vi "Turn Vision.vi"(0 "Angle from camera":dbl, 1 "AUTO ALIGIN":bool, 5 "From Current Pitch Positon":dbl, 7 "From Joystick V Align":dbl, 9 "Angle Gyro":dbl, 10 "True from shooter":bool, 11 "From joystick Right drive":dbl, 12 "From joystick left drive":dbl) -> (4 "To Left Drive":dbl, 6 "To Corrected Pitch":dbl, 8 "To Joystick V Align":dbl, 14 "True to shooter\n(update position)":bool, 15 "To Right Drive":dbl)   [LabVIEW 2015]
uses:
  <vilib>/Rock Robotics/Network Tables/NT Write Boolean.vi
  <vilib>/Rock Robotics/Network Tables/NT Read Number.vi
  <vilib>/Rock Robotics/Network Tables/NT Read Boolean.vi
panel:
  out "Shoot!":bool
  # "From Controller\nFor Vision"
  # "Inputs to controll vision"
  # "Outputs to control robot"
  # "From Controller for no vision"
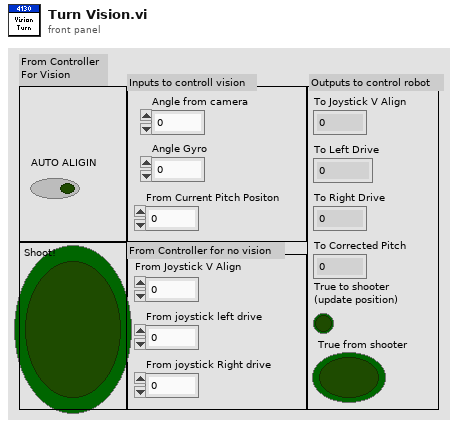
[diagram p1: front panel]
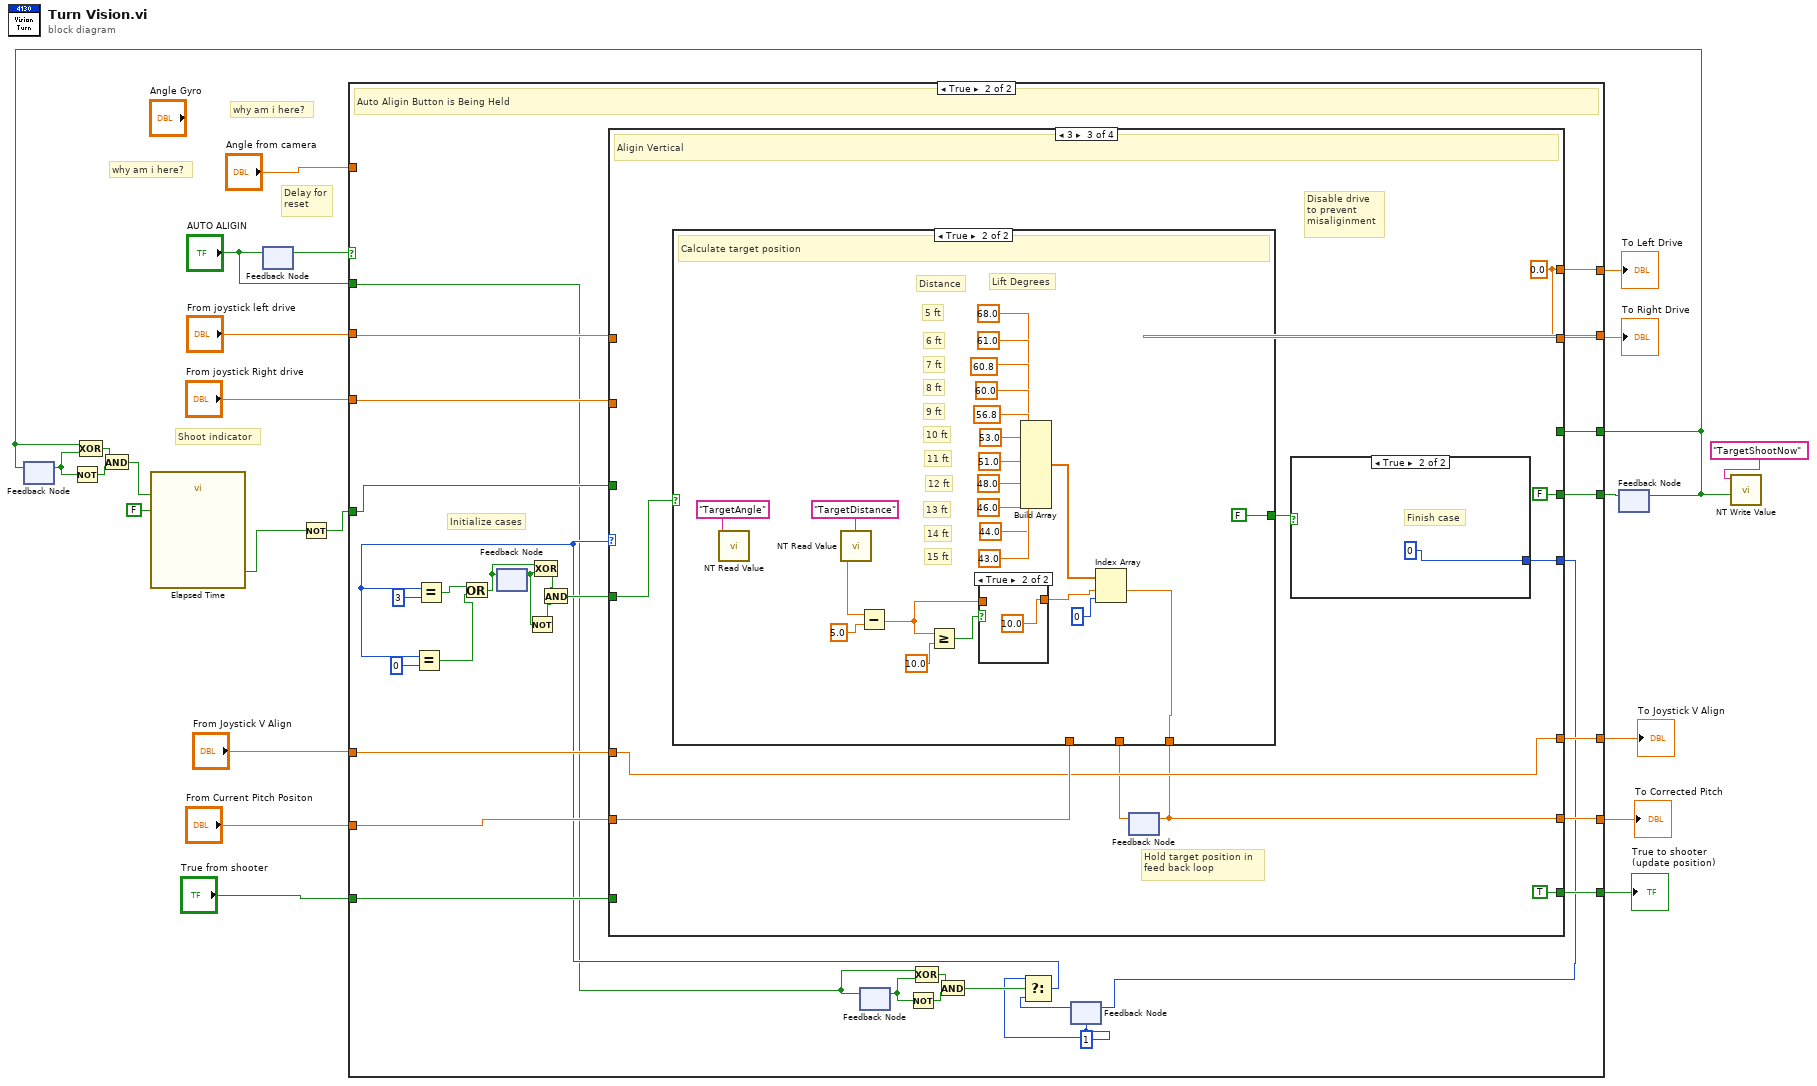
[diagram p0: block diagram]
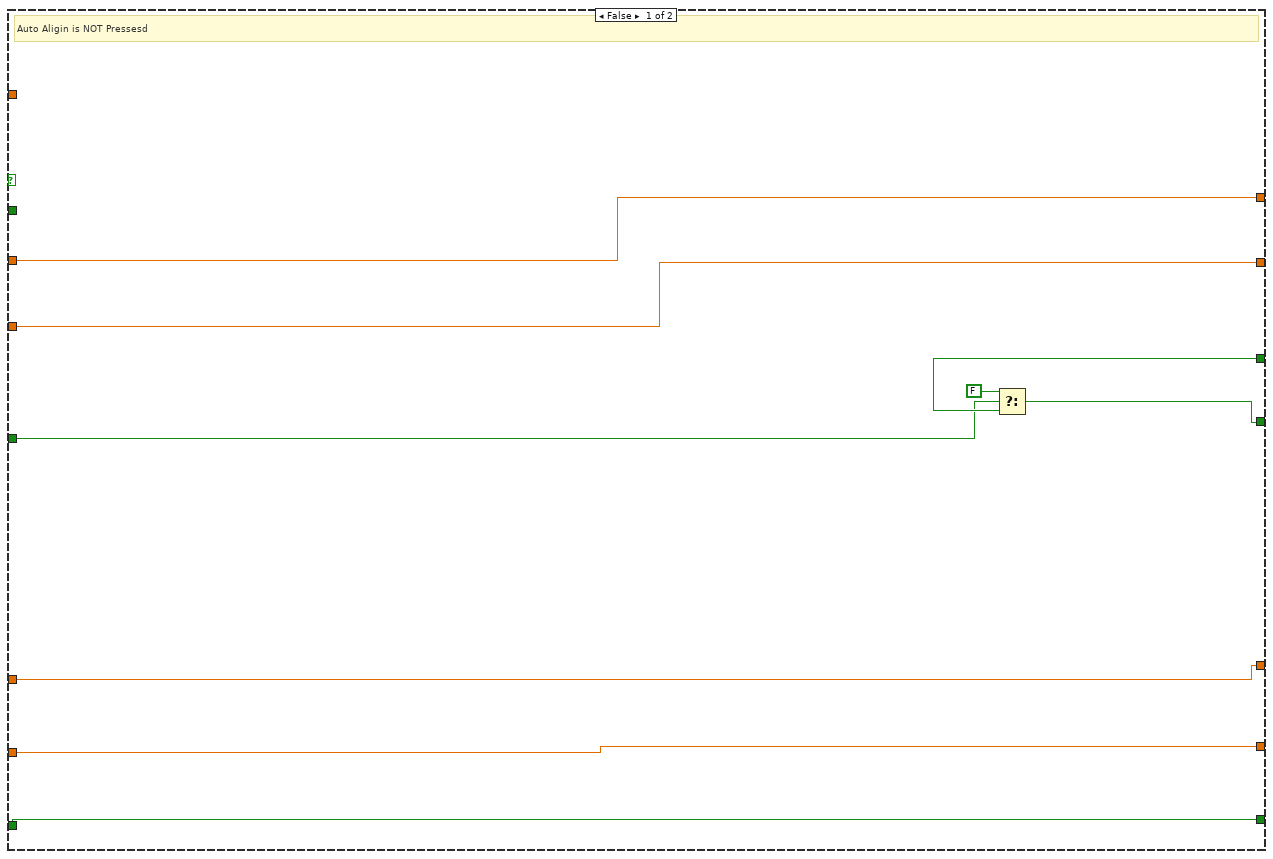
[diagram p2: hidden frame]
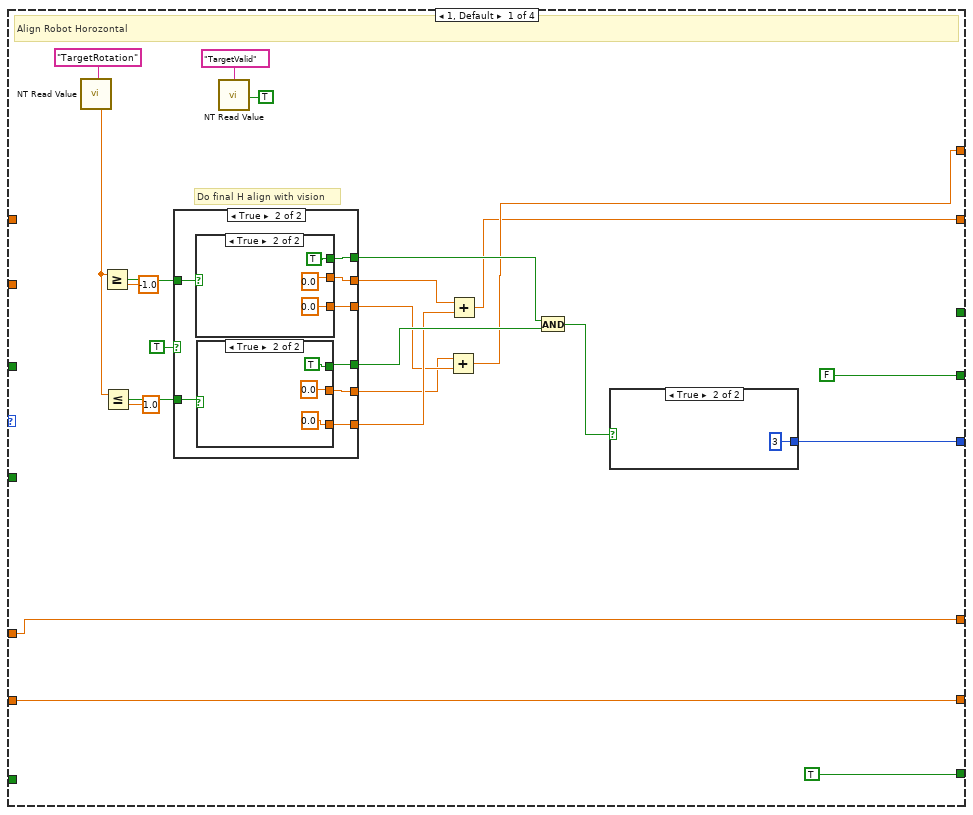
[diagram p3: hidden frame]
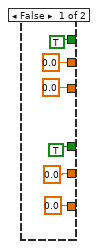
[diagram p4: hidden frame]
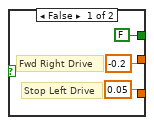
[diagram p5: hidden frame]
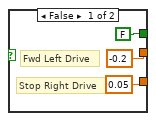
[diagram p6: hidden frame]
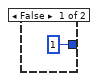
[diagram p7: hidden frame]
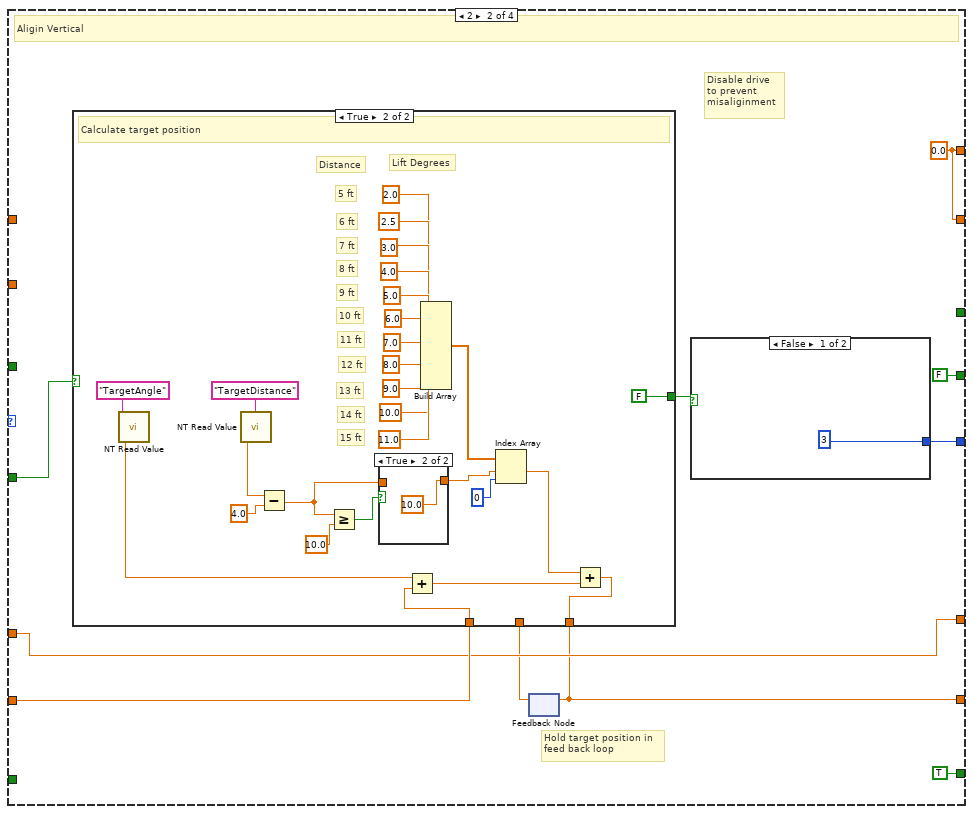
[diagram p8: hidden frame]
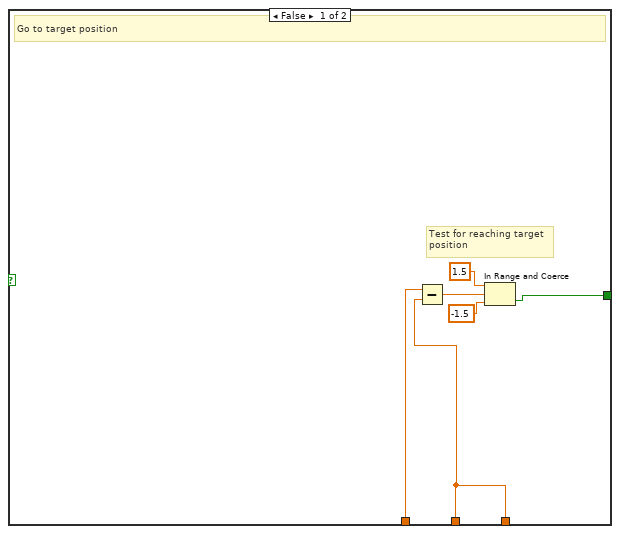
[diagram p9: hidden frame]
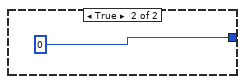
[diagram p11: hidden frame]
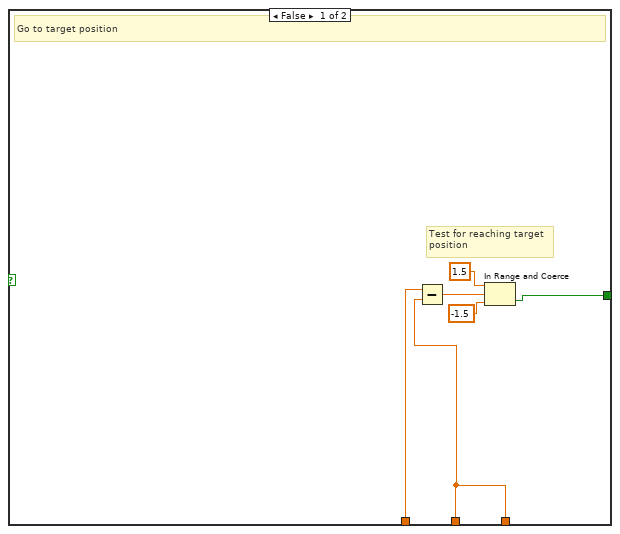
[diagram p12: hidden frame]
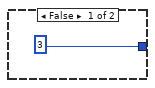
[diagram p14: hidden frame]
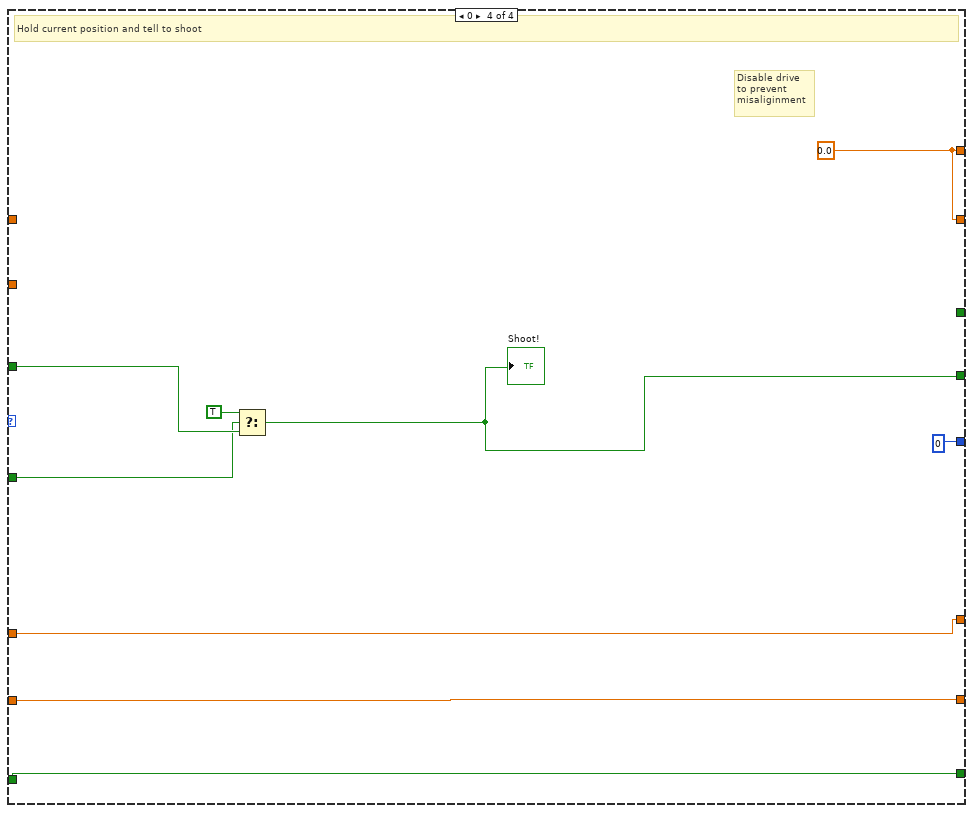
[diagram p15: hidden frame]
diagram:
  # "Shoot indicator"
  # "Delay for\nreset"
  # "why am i here?"
  # "why am i here?"
  n1 = feedback #1() -> (w7:bool)  [unwired: 1 in]
  n2 = Not(x=w7) -> (.not. x?=w9:bool)
  n3 = feedback-in #2("AUTO ALIGIN") -> ()
  n4 = feedback #2() -> (w2:bool)  [unwired: 1 in]
  n5 = feedback #3() -> (w5:bool)  [unwired: 1 in]
  n6 = feedback-in #1(w5) -> ()
  n7 = Compound Arithmetic op=XOR(w5, w7) -> (w8:bool)
  n8 = And(x=w8, y=w9) -> (x .and. y?=w6:bool)
  n9 = call "Elapsed Time"("Reset"=w6, "Auto Reset"=FALSE) -> ("Time has Elapsed"=w4:bool)  [unwired: 10 in, 7 out]
  n10 = Not(x=w4) -> (.not. x?=w3:bool)
  n11 = case shown="True" w2 {
    tunnel: "From joystick Right drive" -> [w32 w58]
    tunnel: "From joystick left drive" -> [w31 w59]
    tunnel: "Angle from camera" -> [_ _]
    tunnel: [w32 w62] -> w22
    tunnel: [w31 w63] -> w23
    tunnel: "From Current Pitch Positon" -> [w30 w61]
    tunnel: [w30 w60] -> w17
    tunnel: "True from shooter" -> [w29 w57]
    tunnel: [w29 w56] -> w15
    tunnel: "From Joystick V Align" -> [w28 w55]
    tunnel: [w28 w54] -> w13
    tunnel: [w27 w43] -> w11
    tunnel: w5 -> [w26 w42]
    tunnel: w3 -> [w24 w41]
    tunnel: "AUTO ALIGIN" -> [_ w36]
    frame False {
      # "Auto Aligin is NOT Pressesd"
      n12 = Select(t=FALSE, s=w24, f=w26) -> (s? t:f=w27:bool)
    }
    frame True {
      w35 = i64 1 ("t")
      # "Initialize cases"
      # "Auto Aligin Button is Being Held"
      n13 = feedback #4() -> (w49:bool)  [unwired: 1 in]
      n14 = Not(x=w49) -> (.not. x?=w47:bool)
      n15 = feedback #5() -> (w51:bool)  [unwired: 1 in]
      n16 = feedback-in #5(w36) -> ()
      n17 = Not(x=w51) -> (.not. x?=w53:bool)
      n18 = Compound Arithmetic op=XOR(w36, w51) -> (w52:bool)
      n19 = And(x=w52, y=w53) -> (x .and. y?=w50:bool)
      n20 = feedback #6(w35) -> (w44:i64)
      n21 = Select(t=w35, s=w50, f=w44) -> (s? t:f=w40:i64)
      n22 = Equal?(x=w40, y=i64 0) -> (x = y?=w37:bool)
      n23 = Equal?(x=w40, y=i64 3) -> (x = y?=w38:bool)
      n24 = Or(x=w38, y=w37) -> (x .or. y?=w39:bool)
      n25 = feedback-in #4(w39) -> ()
      n26 = Compound Arithmetic op=XOR(w39, w49) -> (w48:bool)
      n27 = And(x=w48, y=w47) -> (x .and. y?=w46:bool)
      n28 = case shown="3" w40 {
        tunnel: [w86 w124 w171 i64 0 ("y")] -> w45
        tunnel: [w71 w115 w162 w210] -> w63
        tunnel: [w70 w115 w162 w210] -> w62
        tunnel: w61 -> [w66 w123 w170 w213]
        tunnel: [w66 w118 w165 w213] -> w60
        tunnel: w59 -> [_ _ _ _]
        tunnel: w58 -> [_ _ _ _]
        tunnel: w57 -> [_ _ _ w212]
        tunnel: [TRUE TRUE ("True from shooter") TRUE ("True from shooter") w212] -> w56
        tunnel: w55 -> [w67 w120 w167 w211]
        tunnel: [w67 w120 w167 w211] -> w54
        tunnel: w46 -> [_ w119 w166 w206]
        tunnel: [FALSE FALSE FALSE w208] -> w43
        tunnel: w42 -> [_ _ _ _]
        tunnel: w41 -> [_ _ _ w209]
        frame 1, Default {
          # "Do final H align with vision"
          # "Align Robot Horozontal"
          n29 = call-poly <vilib>:"NT Read Value.vi"("Name"="TargetRotation") -> ("Numeric"=w82:dbl)  [unwired: 9 in, 1 out]
          n30 = Greater Or Equal?(x=w82, y=-1.0) -> (x >= y?=w78:bool)
          n31 = Less Or Equal?(x=w82, y=1.0) -> (x <= y?=w77:bool)
          n32 = case shown="True" TRUE {
            tunnel: [TRUE w100] -> w79
            tunnel: w78 -> [_ w99]
            tunnel: w77 -> [_ w98]
            tunnel: [TRUE w97] -> w76
            tunnel: [0.0 ("y") w96] -> w73
            tunnel: [0.0 ("y") w95] -> w72
            tunnel: [0.0 ("y") w94] -> w74
            tunnel: [0.0 ("y") w93] -> w75
            frame False {
            }
            frame True {
              n33 = case shown="True" w99 {
                tunnel: [-0.2 ("y") 0.0 ("y")] -> w95
                tunnel: [FALSE TRUE] -> w100
                tunnel: [0.05 ("y") 0.0 ("y")] -> w94
                frame False {
                  # "Fwd Left Drive"
                  # "Stop Right Drive"
                }
                frame True {
                }
              }
              n34 = case shown="True" w98 {
                tunnel: [-0.2 ("y") 0.0 ("y")] -> w96
                tunnel: [FALSE TRUE] -> w97
                tunnel: [0.05 ("y") 0.0 ("y")] -> w93
                frame False {
                  # "Fwd Right Drive"
                  # "Stop Left Drive"
                }
                frame True {
                }
              }
            }
          }
          n35 = call-poly <vilib>:"NT Read Value.vi"("Default Value"=TRUE, "Name"="TargetValid") -> ()  [unwired: 8 in, 2 out]
          n36 = Add(x=w73, y=w74) -> (x+y=w71:dbl)
          n37 = Add(x=w72, y=w75) -> (x+y=w70:dbl)
          n38 = And(x=w79, y=w76) -> (x .and. y?=w68:bool)
          n39 = case shown="True" w68 {
            tunnel: [i64 1 ("milliseconds to wait") i64 3 ("milliseconds to wait")] -> w86
            frame False {
            }
            frame True {
            }
          }
        }
        frame 2 {
          w115 = 0.0 ("From joystick left drive")
          # "Disable drive\nto prevent\nmisaliginment"
          # "Hold target position in\nfeed back loop"
          # "Aligin Vertical"
          n40 = feedback #7() -> (w117:dbl)  [unwired: 1 in]
          n41 = case shown="True" w119 {
            tunnel: [w129 w142] -> w118
            tunnel: w123 -> [w130 w136]
            tunnel: [w125 FALSE] -> w122
            tunnel: w117 -> [w129 _]
            frame False {
              # "Test for reaching target\nposition"
              # "Go to target position"
              n42 = Subtract(x=w130, y=w129) -> (x-y=w128:dbl)
              n43 = In Range and Coerce(upper limit=1.5, x=w128, lower limit=-1.5) -> (In Range?=w125:bool)  [unwired: 1 out]
            }
            frame True {
              # "15 ft"
              # "14 ft"
              # "13 ft"
              # "12 ft"
              # "11 ft"
              # "10 ft"
              # "9 ft"
              # "8 ft"
              # "7 ft"
              # "6 ft"
              # "5 ft"
              # "Lift Degrees"
              # "Distance"
              # "Calculate target position"
              n44 = call-poly <vilib>:"NT Read Value.vi"("Name"="TargetAngle") -> ("Numeric"=w134:dbl)  [unwired: 9 in, 1 out]
              n45 = call-poly <vilib>:"NT Read Value.vi"("Name"="TargetDistance") -> ("Numeric"=w145:dbl)  [unwired: 9 in, 1 out]
              n46 = Subtract(x=w145, y=4.0) -> (x-y=w139:dbl)
              n47 = Greater Or Equal?(x=w139, y=10.0) -> (x >= y?=w140:bool)
              n48 = case shown="True" w140 {
                tunnel: [w158 10.0 ("y")] -> w131
                tunnel: w139 -> [w158 _]
                frame False {
                }
                frame True {
                }
              }
              n49 = Add(x=w134, y=w136) -> (x+y=w135:dbl)
              n50 = Build Array(2.0 ("element"), 2.5 ("element"), 3.0 ("element"), 4.0 ("element"), 5.0 ("element"), 6.0 ("element"), 7.0 ("element"), 8.0 ("element"), 9.0 ("element"), 10.0 ("element"), 11.0 ("element")) -> (w133:dbl[])
              n51 = Index Array(array=w133, index #1=w131, index #2=0 ("index")) -> (element #1=w132:dbl)  [unwired: 1 out]
              n52 = Add(x=w132, y=w135) -> (x+y=w142:dbl)
            }
          }
          n53 = feedback-in #7(w118) -> ()
          n54 = case shown="False" w122 {
            tunnel: [i64 3 ("y") i64 0 ("y")] -> w124
            frame False {
            }
            frame True {
            }
          }
        }
        frame 3 {
          w162 = 0.0 ("From joystick left drive")
          # "Disable drive\nto prevent\nmisaliginment"
          # "Hold target position in\nfeed back loop"
          # "Aligin Vertical"
          n55 = feedback #8() -> (w164:dbl)  [unwired: 1 in]
          n56 = case shown="True" w166 {
            tunnel: [w176 w178] -> w165
            tunnel: w170 -> [w177 _]
            tunnel: [w172 FALSE] -> w169
            tunnel: w164 -> [w176 _]
            frame False {
              # "Test for reaching target\nposition"
              # "Go to target position"
              n57 = Subtract(x=w177, y=w176) -> (x-y=w175:dbl)
              n58 = In Range and Coerce(upper limit=1.5, x=w175, lower limit=-1.5) -> (In Range?=w172:bool)  [unwired: 1 out]
            }
            frame True {
              # "15 ft"
              # "14 ft"
              # "13 ft"
              # "12 ft"
              # "11 ft"
              # "10 ft"
              # "9 ft"
              # "8 ft"
              # "7 ft"
              # "6 ft"
              # "5 ft"
              # "Lift Degrees"
              # "Distance"
              # "Calculate target position"
              n59 = call-poly <vilib>:"NT Read Value.vi"("Name"="TargetAngle") -> ()  [unwired: 9 in, 2 out]
              n60 = call-poly <vilib>:"NT Read Value.vi"("Name"="TargetDistance") -> ("Numeric"=w188:dbl)  [unwired: 9 in, 1 out]
              n61 = Subtract(x=w188, y=5.0) -> (x-y=w183:dbl)
              n62 = Greater Or Equal?(x=w183, y=10.0) -> (x >= y?=w184:bool)
              n63 = case shown="True" w184 {
                tunnel: [w201 10.0 ("y")] -> w179
                tunnel: w183 -> [w201 _]
                frame False {
                }
                frame True {
                }
              }
              n64 = Build Array(68.0 ("element"), 61.0 ("element"), 60.8 ("element"), 60.0 ("element"), 56.8 ("element"), 53.0 ("element"), 51.0 ("element"), 48.0 ("element"), 46.0 ("element"), 44.0 ("element"), 43.0 ("element")) -> (w180:dbl[])
              n65 = Index Array(array=w180, index #1=w179, index #2=0 ("index")) -> (element #1=w178:dbl)  [unwired: 1 out]
            }
          }
          n66 = feedback-in #8(w165) -> ()
          n67 = case shown="True" w169 {
            tunnel: [i64 3 ("y") i64 0 ("y")] -> w171
            frame False {
            }
            frame True {
              # "Finish case"
            }
          }
        }
        frame 0 {
          w210 = 0.0 ("From joystick left drive")
          # "Disable drive\nto prevent\nmisaliginment"
          # "Hold current position and tell to shoot"
          n68 = Select(t=TRUE, s=w206, f=w209) -> (s? t:f=w208:bool)
          "Shoot!" <- w208
        }
      }
      n69 = feedback-in #6(w45) -> ()
    }
  }
  "To Left Drive" <- w23
  "To Right Drive" <- w22
  "To Corrected Pitch" <- w17
  "True to shooter\n(update position)" <- w15
  "To Joystick V Align" <- w13
  n70 = feedback-in #3(w11) -> ()
  n71 = call-poly <vilib>:"NT Write Value.vi"("Boolean"=w5, "Name"="TargetShootNow") -> ()  [unwired: 9 in, 1 out]
